vi "launcher.vi"(8 "Error In":errorcluster) -> (0 "Error Out":errorcluster)   [LabVIEW 2018]
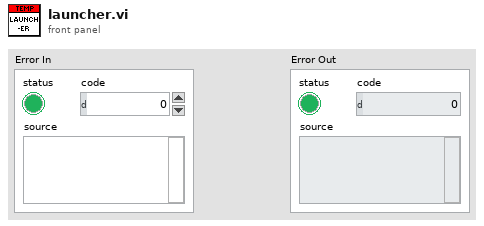
[diagram p1: front panel]
types:
  T1 = enum32{"Invalid", "Standard", "Closed", "Hidden", "Minimized", "Maximized"}
  T2 = typedef "pathCluster.ctl" = cluster{"src Folder Path":path, "Controller Module Path":path, "UI Module Path":path, "Model Select Module Path":path, "Barcode Printer Module Path":path, "Barcode Scanner Module Path":path, "Database Module Path":path, "Report Generation Path":path, "Simulation Path":path, "subVIs Folder Path":path, "info Folder Path":path, "config file Path":path, "cutomerLogo Path":path, "database File Path":path}
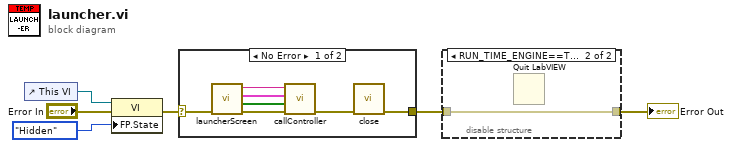
[diagram p0: block diagram]
diagram:
  n1 = control-ref of="This VI"() -> (w4:refnum<vi>)
  n2 = property class="VI"(reference=w4, error in="Error In", "FP.State"=T1."Hidden" ("Front Panel Window:State")) -> (error out=w1:errorcluster)  [unwired: 1 out]
  n3 = case shown="No Error" w1 {
    selector: w1 -> [w13 w14]
    tunnel: [w12 w14] -> w6
    frame No Error {
      n4 = call "launcherScreen.vi"("Error In"=w13) -> ("Error Out"=w11:errorcluster, "simulationModule"=w7:bool[], "Application Path Cluster"=w8:T2, "Software Name"=w9:string)  [unwired: 7 in]
      n5 = call "callController.vi"("Error In"=w11, "Simulation Module"=w7, "Application Path Cluster"=w8, "Software Name"=w9) -> ("Error Out"=w10:errorcluster)  [unwired: 7 in]
      n6 = call "close.vi"("error in (no error)"=w10) -> ("error out"=w12:errorcluster)  [unwired: 10 in]
    }
    frame Error {
    }
  }
  n7 = disable-structure shown="RUN_TIME_ENGINE==True" {
    disable-tunnel: w6 -> [w15 w16]
    disable-tunnel: [w15 w16] -> w5
    frame condition #0 (active) {
    }
    frame condition #1 {
      n8 = Quit LabVIEW() -> ()  [unwired: 1 in]
    }
  }
  "Error Out" <- w5
